vi "Remote1Button11.vi"() -> (0 "Pressed?":bool)   [LabVIEW 2010, in "FTC.lvlib" / "Remote Interface.lvlib"]
uses:
  Remote Interface.lvlib
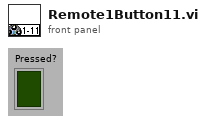
[diagram p1: front panel]
types:
  T1 = enum16{"1-1", "1-2", "1-3", "1-4", "1-5", "1-6", "1-7", "1-8", "1-9", "1-10", "1-11", "1-12", "2-1", "2-2", "2-3", "2-4", "2-5", "2-6", "2-7", "2-8", "2-9", "2-10", "2-11", "2-12", "NXT-L", "NXT-R", "NXT-E"}
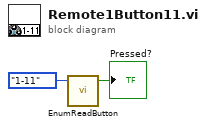
[diagram p0: block diagram]
diagram:
  n1 = call "EnumReadButton.vi"("Button"=T1."1-11") -> ("Pressed?"=→"Pressed?":bool)  [unwired: 4 in]
